vi "Exp_Test 2.vi"(0 "object in":refnum<class "SaveData.lvclass">, 2 "output cluster":T2, 3 "Temperature(C)":dbl, 4 "Oscilloscope Results 2":T1 {"Probe Current" format="%.2p"; "Phase Angle" format="%.2p"; "Main Freq" format="%.2p"; "Main Volt" format="%.2p"}, 5 "error in (no error)":errorcluster) -> (14 "object out":refnum<class "SaveData.lvclass">, 19 "error out":errorcluster)   [LabVIEW 2023, in "SaveData.lvclass"]
uses:
  SaveData.lvclass
  SaveData.lvclass/SaveData.ctl
  <vilib>/express/express shared/transition.llb/Dynamic To Waveform Array.vi
  <vilib>/express/express signal manip/GetorSetDDTAttributes/Set DDT Attributes/SetT0.vi
  <vilib>/express/express shared/transition.llb/Waveform Array To Dynamic.vi
  <vilib>/express/express signal manip/GetorSetDDTAttributes/Set DDT Attributes/Set DDT Properties.xnode
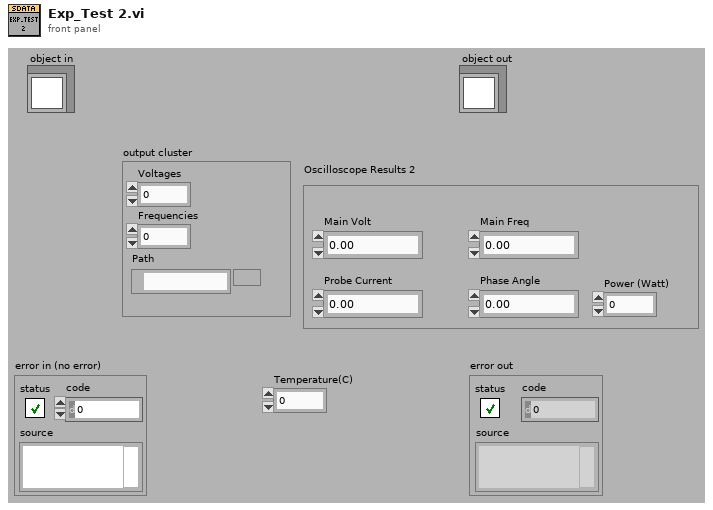
[diagram p1: front panel]
types:
  T1 = cluster{"Main Volt":dbl, "Main Freq":dbl, "Phase Angle":dbl, "Probe Current":dbl, "Power (Watt)":dbl}
  T2 = cluster{"Voltages":dbl, "Frequencies":dbl, "Path":path}
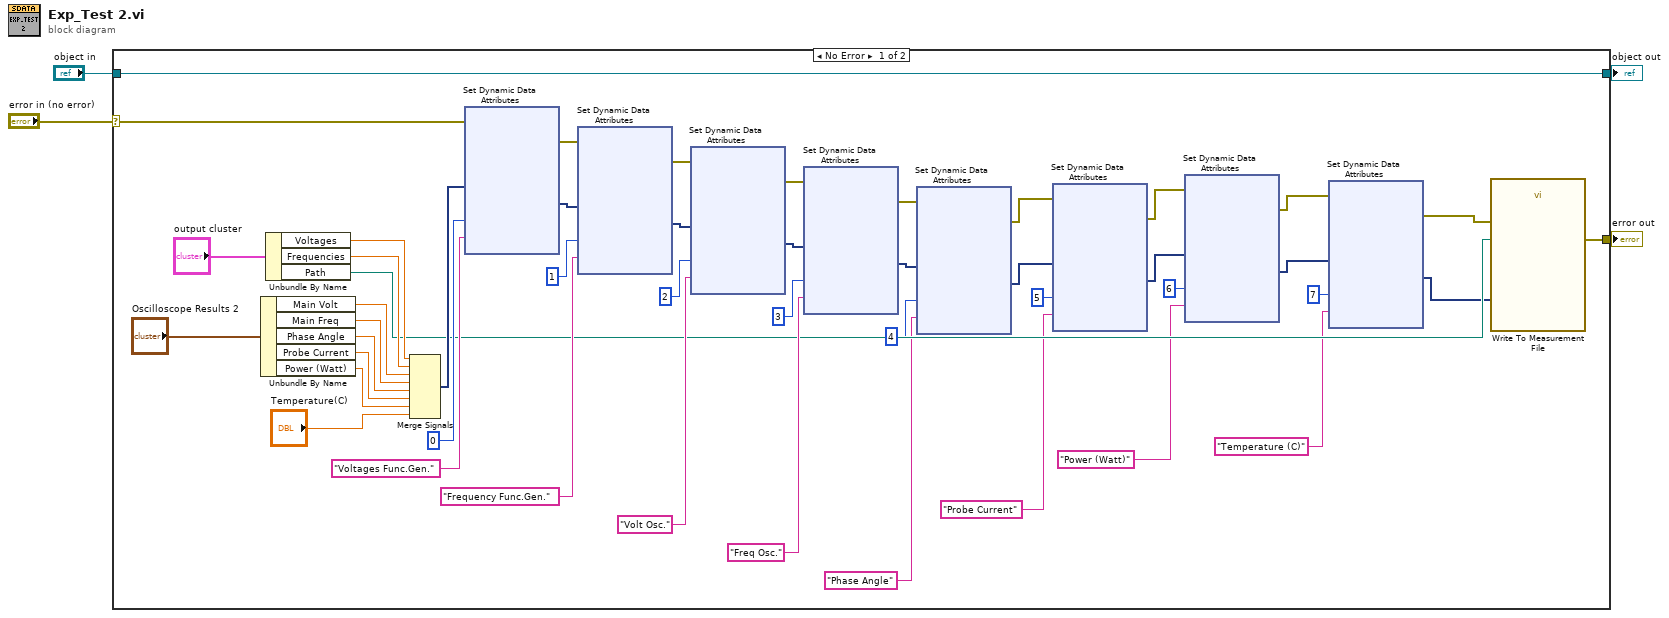
[diagram p0: block diagram]
diagram:
  n1 = case shown="No Error" "error in (no error)" {
    selector: "error in (no error)" -> [w24 w157]
    tunnel: [w25 w157] -> w3
    tunnel: [w51 w156] -> w1
    tunnel: "object in" -> [w51 w156]
    frame No Error {
      n2 = Unbundle By Name("Oscilloscope Results 2") -> ("Main Volt"=w34:dbl, "Main Freq"=w33:dbl, "Phase Angle"=w30:dbl, "Probe Current"=w21:dbl, "Power (Watt)"=w20:dbl)
      n3 = Unbundle By Name("output cluster") -> ("Voltages"=w36:dbl, "Frequencies"=w35:dbl, "Path"=w31:path)
      n4 = Merge Signals(w36, w35, w34, w33, w30, w21, w20, "Temperature(C)") -> (w32:dynamicdata)
      n5 = xnode "Set Dynamic Data Attributes"("Signals In"=w32, "Signal Index"=0, "Signal Name"="Voltages Func.Gen.", "error in"=w24) -> ("Signals Out"=w39:dynamicdata, "error out"=w48:errorcluster)
      n6 = xnode "Set Dynamic Data Attributes"("Signals In"=w39, "Signal Index"=1, "Signal Name"="Frequency Func.Gen.", "error in"=w48) -> ("Signals Out"=w38:dynamicdata, "error out"=w47:errorcluster)
      n7 = xnode "Set Dynamic Data Attributes"("Signals In"=w38, "Signal Index"=2, "Signal Name"="Volt Osc.", "error in"=w47) -> ("Signals Out"=w37:dynamicdata, "error out"=w46:errorcluster)
      n8 = xnode "Set Dynamic Data Attributes"("Signals In"=w37, "Signal Index"=3, "Signal Name"="Freq Osc.", "error in"=w46) -> ("Signals Out"=w28:dynamicdata, "error out"=w29:errorcluster)
      n9 = xnode "Set Dynamic Data Attributes"("Signals In"=w28, "Signal Index"=4, "Signal Name"="Phase Angle", "error in"=w29) -> ("Signals Out"=w14:dynamicdata, "error out"=w18:errorcluster)
      n10 = xnode "Set Dynamic Data Attributes"("Signals In"=w14, "Signal Index"=5, "Signal Name"="Probe Current", "error in"=w18) -> ("Signals Out"=w13:dynamicdata, "error out"=w17:errorcluster)
      n11 = xnode "Set Dynamic Data Attributes"("Signals In"=w13, "Signal Index"=6, "Signal Name"="Power (Watt)", "error in"=w17) -> ("Signals Out"=w12:dynamicdata, "error out"=w16:errorcluster)
      n12 = xnode "Set Dynamic Data Attributes"("Signals In"=w12, "Signal Index"=7, "Signal Name"="Temperature (C)", "error in"=w16) -> ("Signals Out"=w8:dynamicdata, "error out"=w15:errorcluster)
      n13 = call "Write To Measurement File"("Signals"=w8, "error in (no error)"=w15, "Filename"=w31) -> ("error out"=w25:errorcluster)  [unwired: 14 in, 2 out]
    }
    frame Error {
    }
  }
  "error out" <- w3
  "object out" <- w1
